vi "NF LI56xx dvr DATA FEED CONTrol.vi"(8 "error in":errorcluster caption="error in (no error)" {"code" format="%.0x"}, 9 "Read(F)":bool, 10 "set buffer":enum16{"BUF1", "BUF2", "BUF3"}(ring), 11 "VISA resource name":refnum<visa-resource-name>) -> (0 "error out":errorcluster {"code" format="%.0x"}, 2 "query data recording type":string, 3 "VISA resource name copy":refnum<visa-resource-name>)   [LabVIEW 2019]
doc: "Sets/queries whether measurement data is to be recorded in a measurement data buffer."
panel:
  in  "set data recording type":enum16{"ALWays", "NEVer"}(ring)
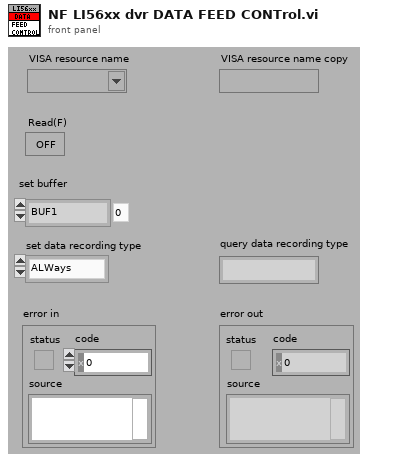
[diagram p1: front panel]
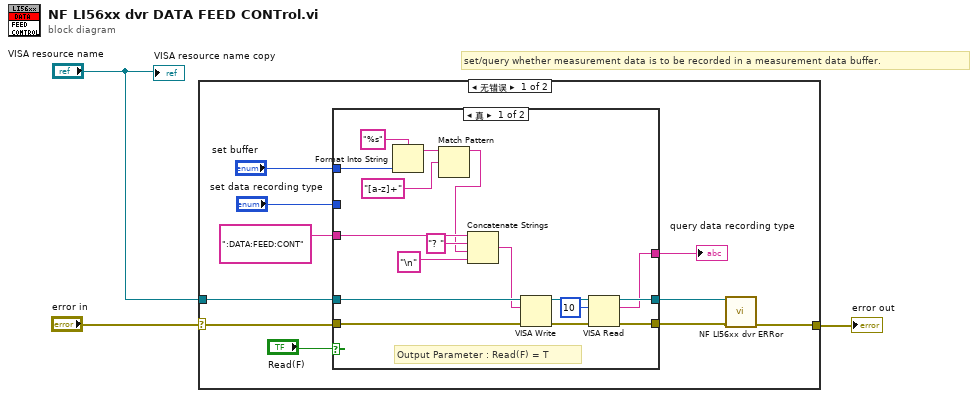
[diagram p0: block diagram]
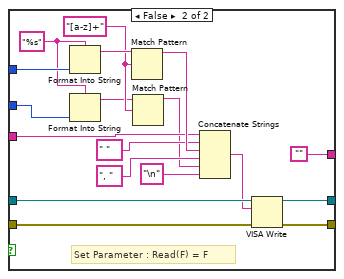
[diagram p2: hidden frame]
diagram:
  # "set/query whether measurement data is to be recorded in a measurement data buffer."
  n1 = case shown="无错误" "error in" {
    selector: "error in" -> [w12 w49]
    tunnel: [w6 w49] -> w3
    tunnel: "VISA resource name" -> [w11 _]
    frame No Error {
      n2 = case shown="真" "Read(F)" {
        tunnel: w11 -> [w30 w48]
        tunnel: [w27 w45] -> w8
        tunnel: [w26 w46] -> w7
        tunnel: w12 -> [w25 w47]
        tunnel: [w21 ""] -> w10
        tunnel: "set buffer" -> [w16 w42]
        tunnel: ":DATA:FEED:CONT" ("•¶Žš—ñ") -> [w20 w39]
        tunnel: "set data recording type" -> [_ w31]
        frame True {
          # "Output Parameter : Read(F) = T"
          n3 = Format Into String(format string="%s", w16) -> (resulting string=w18:string)  [unwired: 2 in, 1 out]
          n4 = Match Pattern(string=w18, regular expression="[a-z]+") -> (before substring=w15:string)  [unwired: 1 in, 3 out]
          n5 = Concatenate Strings(w20, "? " ("Œ`Ž®•¶Žš—ñ"), w15, "\n" ("Œ`Ž®•¶Žš—ñ")) -> (w22:string)
          n6 = VISA Write(VISA resource name=w30, write buffer=w22, error in (no error)=w25) -> (VISA resource name out=w28:refnum<visa-resource-name>, error out=w29:errorcluster)  [unwired: 1 out]
          n7 = VISA Read(VISA resource name=w28, byte count=u32 10 ("バイトカウント（0）"), error in (no error)=w29) -> (VISA resource name out=w27:refnum<visa-resource-name>, read buffer=w21:string, error out=w26:errorcluster)  [unwired: 1 out]
        }
        frame False {
          w34 = "[a-z]+"
          w32 = "%s"
          # "Set Parameter : Read(F) = F"
          n8 = Format Into String(format string=w32, w42) -> (resulting string=w41:string)  [unwired: 2 in, 1 out]
          n9 = Format Into String(format string=w32, w31) -> (resulting string=w33:string)  [unwired: 2 in, 1 out]
          n10 = Match Pattern(string=w41, regular expression=w34) -> (before substring=w40:string)  [unwired: 1 in, 3 out]
          n11 = Match Pattern(string=w33, regular expression=w34) -> (before substring=w35:string)  [unwired: 1 in, 3 out]
          n12 = Concatenate Strings(w39, " ", w40, ", ", w35, "\n" ("Œ`Ž®•¶Žš—ñ")) -> (w43:string)
          n13 = VISA Write(VISA resource name=w48, write buffer=w43, error in (no error)=w47) -> (VISA resource name out=w45:refnum<visa-resource-name>, error out=w46:errorcluster)  [unwired: 1 out]
        }
      }
      "query data recording type" <- w10
      n14 = call "NF LI56xx dvr ERRor.vi"("VISA resource name"=w8, "error in (no error)"=w7) -> ("error out"=w6:errorcluster)  [unwired: 10 in, 3 out]
    }
    frame Error {
    }
  }
  "error out" <- w3
  "VISA resource name copy" <- "VISA resource name"
